vi "ITX to PG.vi"(6 "Numeric":i32, 8 "error in (no error)":errorcluster, 11 "Path":path) -> (0 "error out":errorcluster, 2 "Not Equal?":bool, 3 "Path out":path, 5 "Data out":refnum<class "Data.lvclass">)   [LabVIEW 2016]
uses:
  Data/Data.lvclass
  Data/Typedefs/File Type--enum.ctl
  Data/Typedefs/Operation--enum.ctl
  Data/Typedefs/Dictionary--cluster.ctl
panel:
  out "Dictionary":T1[](array[typedef])
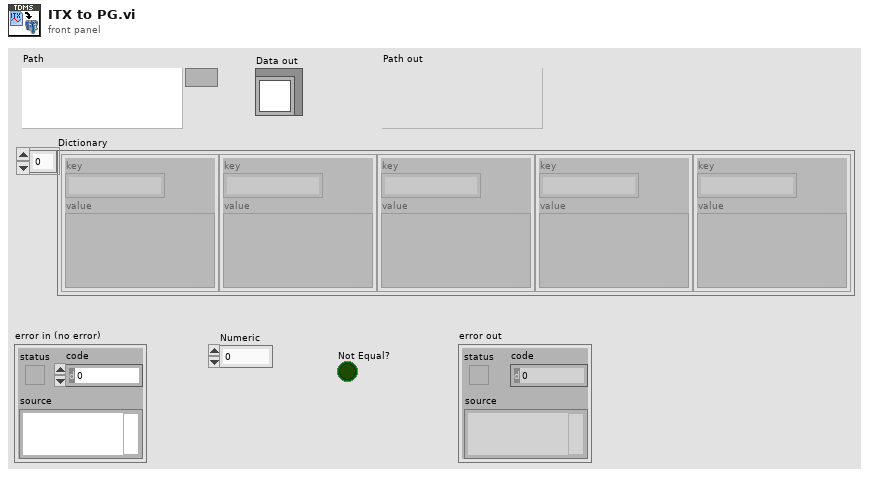
[diagram p1: front panel]
types:
  T1 = typedef "Data.lvclass/Dictionary--cluster.ctl" = cluster{"key":string, "value":variant}
  T2 = typedef "Data.lvclass/File Type--enum.ctl" = enum16{"DAT", "ITX", "HDF5", "TDMS", "VI", "PGSQL"}
  T3 = typedef "Data.lvclass/Operation--enum.ctl" = enum16{"Read", "Write", "Write + Append"}
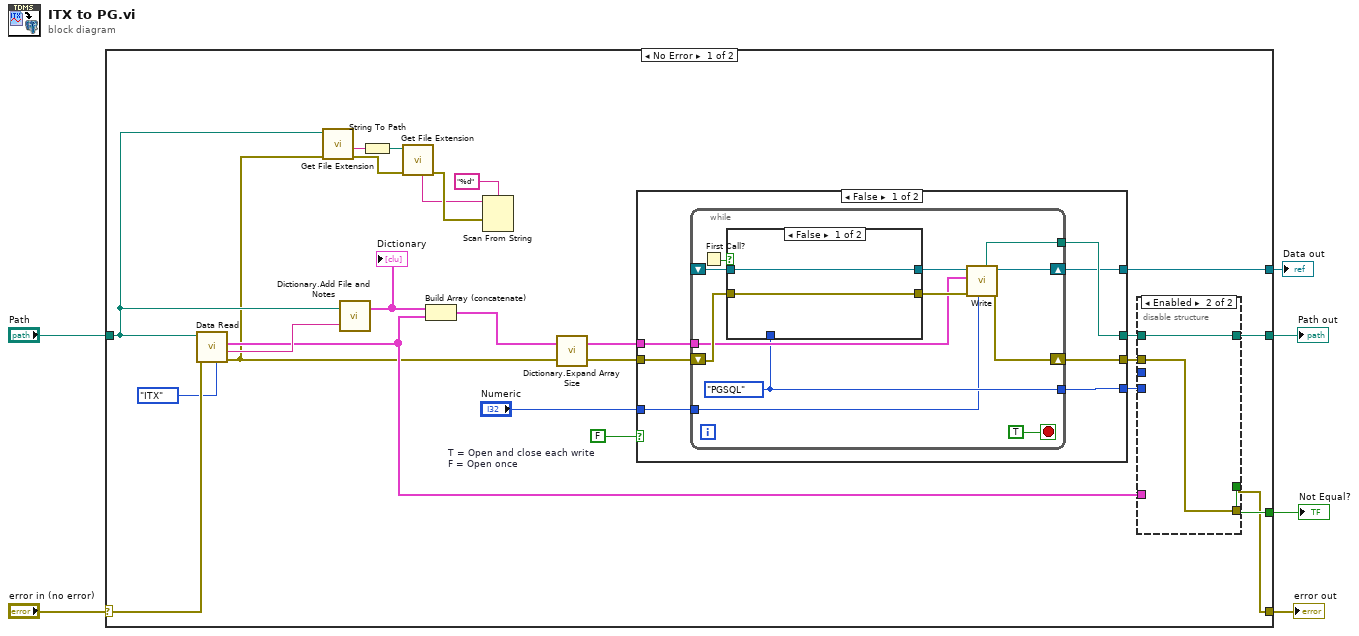
[diagram p0: block diagram]
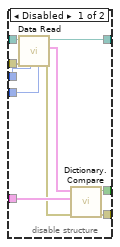
[diagram p2: hidden frame]
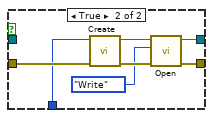
[diagram p3: hidden frame]
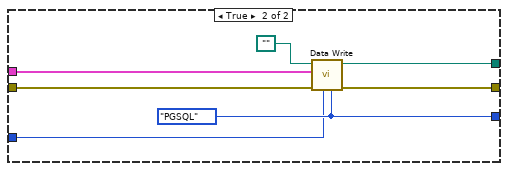
[diagram p4: hidden frame]
diagram:
  n1 = case shown="No Error" "error in (no error)" {
    selector: "error in (no error)" -> [w31 w79]
    tunnel: [w26 w79] -> w5
    tunnel: "Path" -> [w9 _]
    tunnel: [w28 _] -> w3
    tunnel: [w27 _] -> w2
    tunnel: [w23 _] -> w1
    frame No Error {
      w22 = FALSE  # T = Open and close each write F = Open once
      n2 = call "Data Read.vi"("File Type"=File_Type--enum."ITX", "error in (no error)"=w31, "path"=w9) -> ("error out"=w8:errorcluster, "Notes"=w19:string, "Data (Dictionary)"=w16:T1[])  [unwired: 5 in, 1 out]
      n3 = call <vilib>:"Get File Extension.vi"("error in (no error)"=w8, "file"=w9) -> ("error out"=w13:errorcluster, "filename without extension"=w14:string)  [unwired: 8 out]
      n4 = call "Dictionary.Add File and Notes.vi"("Notes"=w19, "Path"=w9) -> ("Dictionary"=w18:T1[])  [unwired: 1 in]
      "Dictionary" <- w18
      n5 = String To Path(string=w14) -> (path=w15:path)
      n6 = call <vilib>:"Get File Extension.vi"("error in (no error)"=w13, "file"=w15) -> ("error out"=w11:errorcluster, "unmodified file extension"=w10:string)  [unwired: 8 out]
      n7 = Build Array (concatenate)(w18, w16) -> (w17:T1[])
      n8 = Scan From String(format string="%d", input string=w10, error in=w11) -> ()  [unwired: 3 in, 3 out]
      n9 = call "Dictionary.Expand Array Size.vi"("error in (no error)"=w8, "Data (Dictionary)"=w17) -> ("error out"=w20:errorcluster, "Dictionary"=w21:T1[])
      n10 = case shown="False" w22 {
        tunnel: [w46 w78] -> w30
        tunnel: [w49 w77] -> w29
        tunnel: w21 -> [w48 w76]
        tunnel: w20 -> [w50 w75]
        tunnel: [w47 w74] -> w25
        tunnel: [w45 _] -> w23
        tunnel: "Numeric" -> [w44 w72]
        frame False {
          n11 = while {
            tunnel: w48 -> [w58]
            tunnel: [w54] -> w47
            shift-right: [w59] -> w49
            shift-left: w50 -> [w60]
            shift-right: [w57] -> w45
            shift-left: _ -> [w55]
            tunnel: [w52] -> w46
            tunnel: w44 -> [w51]
            stop <- TRUE stop-if-true
            w54 = File_Type--enum."PGSQL" ("File Type")
            n12 = First Call?() -> (First Call?: T/F=w56:bool)
            n13 = case shown="False" w56 {
              tunnel: [w63 w71] -> w62
              tunnel: [w64 w70] -> w61
              tunnel: w60 -> [w63 w67]
              tunnel: w54 -> [_ w66]
              tunnel: w55 -> [w64 _]
              frame False {
              }
              frame True {
                n14 = call "Create.vi"("error in (no error)"=w67, "File Type"=w66) -> ("error out"=w68:errorcluster, "Data out"=w69:refnum<class "Data.lvclass">)  [unwired: 8 in]
                n15 = call-dynamic "Open.vi"("error in (no error)"=w68, "Operation"=Operation--enum."Write", "Data in"=w69) -> ("error out"=w71:errorcluster, "Data out"=w70:refnum<class "Data.lvclass">)  [unwired: 7 in]
              }
            }
            n16 = call-dynamic "Write.vi"("Append Index"=w51, "error in (no error)"=w62, "Data (Dictionary)"=w58, "Data in"=w61) -> ("error out"=w59:errorcluster, "Data out"=w57:refnum<class "Data.lvclass">, "Path out"=w52:path)  [unwired: 5 in]
          }
        }
        frame True {
          w74 = File_Type--enum."PGSQL" ("File Type")
          n17 = call "Data Write.vi"("File Type"=w74, "Append Index"=w72, "error in (no error)"=w75, "Data (Dictionary)"=w76, "path"=path "") -> ("error out"=w77:errorcluster, "path out"=w78:path)  [unwired: 5 in]
        }
      }
      n18 = disable-structure shown="Enabled" {
        disable-tunnel: w30 -> [w41 w42]
        disable-tunnel: w29 -> [w40 w43]
        disable-tunnel: [w39 w42] -> w28
        disable-tunnel: w16 -> [w37 _]
        disable-tunnel: [w36 _] -> w27
        disable-tunnel: [w34 w43] -> w26
        disable-tunnel: w25 -> [w33 _]
        disable-tunnel: _ -> [w32 _]
        frame Disabled {
          n19 = call "Data Read.vi"("File Type"=w33, "Append Index"=w32, "error in (no error)"=w40, "path"=w41) -> ("error out"=w35:errorcluster, "Data (Dictionary)"=w38:T1[], "path out"=w39:path)  [unwired: 4 in, 1 out]
          n20 = call "Dictionary.Compare.vi"("error in (no error)"=w35, "Original Data (Dictionary)"=w37, "Converted Data (Dictionary)"=w38) -> ("error out"=w34:errorcluster, "Not Equal?"=w36:bool)  [unwired: 7 in]
        }
        frame Enabled {
        }
      }
    }
    frame Error {
    }
  }
  "error out" <- w5
  "Path out" <- w3
  "Not Equal?" <- w2
  "Data out" <- w1
